vi "Signals.Get.vi"(8 "error in (no error)":errorcluster, 11 "Device Item Ref out":T1 format="%.0x") -> (0 "error out":errorcluster, 1 "Parameters":T2[](array[typedef]) {"Byte Order" items=["Little Endian", "Big Endian"]; "Data Type" items=["Signed", "Unsigned", "IEEE Float"]}, 2 "Child Refs":T1[](array[typedef]) format="%.0x", 3 "Item Ref out":T1 format="%.0x")   [LabVIEW 2019, in "Diagnostics Addon System Explorer.lvlib"]
uses:
  Diagnostics Addon System Explorer.lvlib
  <vilib>/NI VeriStand/Custom Device API/Custom Device Item Ref.ctl
  Addon Shared/Types/Signal.ctl
  Types/FG.Action.ctl
  Addon Shared/SubVIs/Constants.vi
  <vilib>/NI VeriStand/Custom Device API/NI VeriStand - Get Item Data.vi
  <vilib>/NI VeriStand/Custom Device Tools/Custom Device Utility Library/NI VeriStand - Search for Item.vi
  <vilib>/NI VeriStand/Custom Device Tools/Custom Device Utility Library/NI VeriStand - Search for Item by GUID.vi
  <vilib>/NI VeriStand/Custom Device API/NI VeriStand - Get Item Children.vi
  <vilib>/NI/NI VeriStand Advanced SysDef API/SysDef API/SysDef.Property.Set.vi
  <vilib>/NI/NI VeriStand Advanced SysDef API/_SubVIs/SysDef.Property.Set.U32.vi
  <vilib>/NI/NI VeriStand Advanced SysDef API/_SubVIs/SysDef.Property.Set.DBL.vi
  <vilib>/NI/NI VeriStand Advanced SysDef API/_SubVIs/SysDef.Property.Set.String.vi
  <vilib>/NI VeriStand/Custom Device API/NI VeriStand - Get Item Property.vi
  <vilib>/NI VeriStand/Custom Device API/Get Item Property (U32).vi
  <vilib>/NI VeriStand/Custom Device API/Get Item Property (Double).vi
  <vilib>/NI VeriStand/Custom Device API/Get Item Property (String).vi
  <vilib>/NI VeriStand/Custom Device API/Custom Device API.lvlib
  Addon Shared/Diagnostics Addon Shared.lvlib
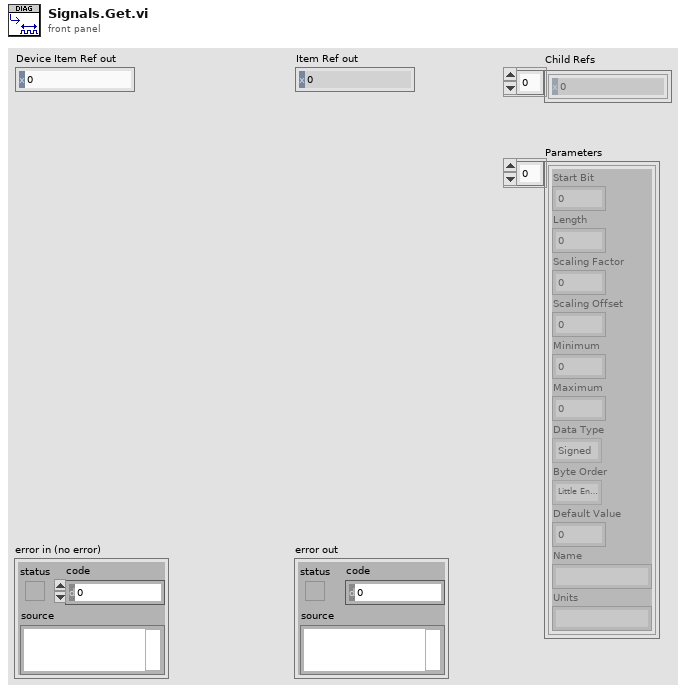
[diagram p1: front panel]
types:
  T1 = typedef "Custom Device API.lvlib/Custom Device Item Ref.ctl" = u64
  T2 = typedef "Diagnostics Addon Shared.lvlib/Signal.ctl" = cluster{"Start Bit":u32, "Length":u32, "Scaling Factor":dbl, "Scaling Offset":dbl, "Minimum":dbl, "Maximum":dbl, "Data Type":u32, "Byte Order":u32, "Default Value":dbl, "Name":string, "Units":string}
  T3 = typedef "Diagnostics Addon System Explorer.lvlib/FG.Action.ctl" = enum16{"Get", "Set"}
  T4 = typedef "Custom Device API.lvlib/Custom Device Channel.ctl" = cluster{"Type":T5, "Units":string, "Default Value":dbl, "Faultable":bool, "Scalable":bool}
  T5 = typedef "Custom Device API.lvlib/Custom Device Channel Type.ctl" = enum16{"Input", "Output"}
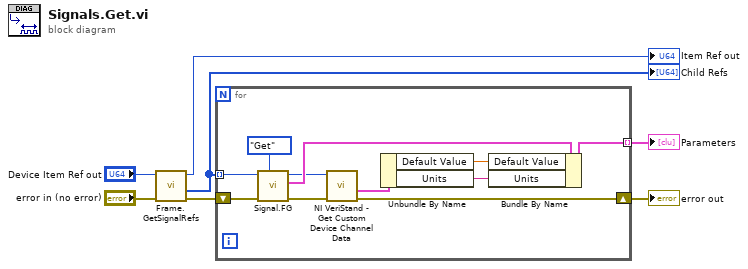
[diagram p0: block diagram]
diagram:
  n1 = call "Frame.GetSignalRefs.vi"("error in (no error)"="error in (no error)", "Frame Item Ref in"="Device Item Ref out") -> ("error out"=w6:errorcluster, "Child Refs"=w1:T1[], "Original Frame Ref out"=→"Item Ref out":T1)  [unwired: 6 in, 1 out]
  "Child Refs" <- w1
  n2 = for {
    shift-right: [w18] -> w7
    shift-left: w6 -> [w11]
    tunnel: w1 -> [w10] mode=indexing
    tunnel: [w17] -> w5 mode=indexing
    n3 = call "Signal.FG.vi"("Action"=FG.Action."Get", "error in (no error)"=w11, "Device Item Ref in"=w10) -> ("error out"=w9:errorcluster, "Signal Parameters"=w16:T2, "Device Item Ref out"=w8:T1)  [unwired: 6 in]
    n4 = call <vilib>:"NI VeriStand - Get Custom Device Channel Data.vi"("error in (no error)"=w9, "Channel Ref in"=w8) -> ("error out"=w18:errorcluster, "Channel"=w15:T4)  [unwired: 4 in, 4 out]
    n5 = Unbundle By Name(w15) -> ("Default Value"=w13:dbl, "Units"=w14:string)
    n6 = Bundle By Name(cluster=w16, "Default Value"=w13, "Units"=w14) -> (w17:T2)
  }
  "error out" <- w7
  "Parameters" <- w5
